vi "SIDKSID4_UtilsSDK_StringLengthMax.vi"() -> (0 "lgeur max chaine char":u32)   [LabVIEW 2013]
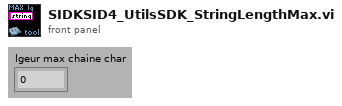
[diagram p1: front panel]
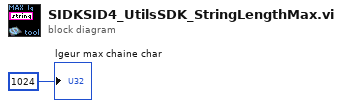
[diagram p0: block diagram]
diagram:
  "lgeur max chaine char" <- u32 1024
